vi "IMAQ FPGA Camera Link Pixel Bus to Vision Pixel Bus U32x1.vi"(5 "Reset Overflow":bool, 6 "Ready for Output":bool=TRUE, 7 "Overflow In":bool, 8 "Input Valid":bool=TRUE, 9 "Frame Valid In":bool, 10 "Line Valid In":bool, 11 "Pixel In":u32) -> (0 "Output Valid":bool, 2 "Acquisition Overflow":bool, 3 "Vision Pixel Bus Out":T1)   [LabVIEW 2020]
doc: "The Pixel Bus to Vision Pixel Bus takes the <B>Pixel In</B> and the timing signals (Line Valid, Frame Valid, and Input Valid) and converts them to the data structure used by Vision FPGA functions where the Line Valid and Frame Valid are part of the <B>Vision Pixel Bus Out</B> data structure.\n\nIf Ready For Output is ever False (i.e. downstream VIs are not ready for new pixel data), and this VI is about to output a valid Vision Pixel Bus, the Acquisition Overflow will assert and stay high to indicate pixel data was lost. The CameraLink pixel bus can not be slowed down, so the downstream processing VIs and transfer VIs need to ensure they can handle the CameraLink throughput to avoid missing pixels."
uses:
  <vilib>/visionFPGA/Controls/IMAQ FPGA Pixel Bus RGB32x1.ctl
  <vilib>/visionFPGA/Basics/Camera Link Acquisition/Controls/IMAQ FPGA Camera Link Pixel Bus to Vision Bus State.ctl
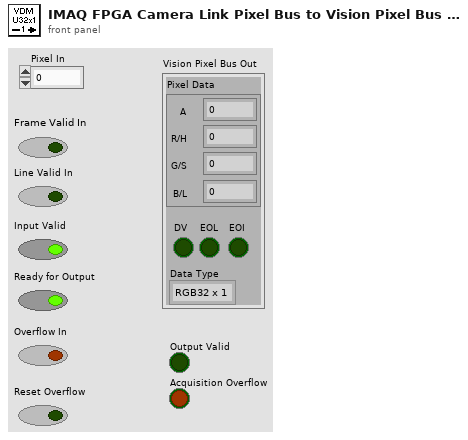
[diagram p1: front panel]
types:
  T1 = typedef "IMAQ FPGA Pixel Bus RGB32x1.ctl" = cluster{"Pixel Data":cluster{"A":u8, "R/H":u8, "G/S":u8, "B/L":u8}, "DV":bool, "EOL":bool, "EOI":bool, "Data Type":enum16{"RGB32 x 1"}}
  T2 = typedef "IMAQ FPGA Camera Link Pixel Bus to Vision Bus State.ctl" = enum16{"WaitForFirstPixel", "WaitForEndOfLine", "WaitForStartofNextLineOrEndOfImage", "HandleEndOfImage"}
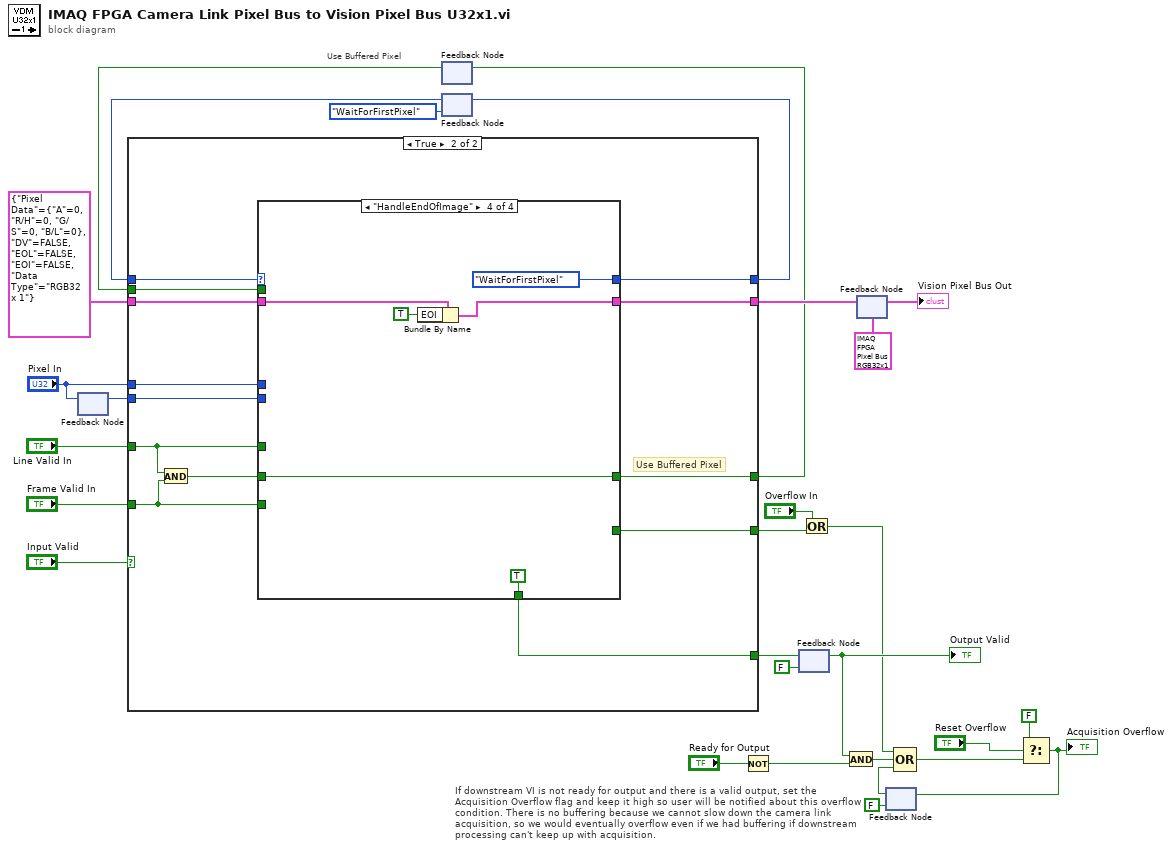
[diagram p0: block diagram]
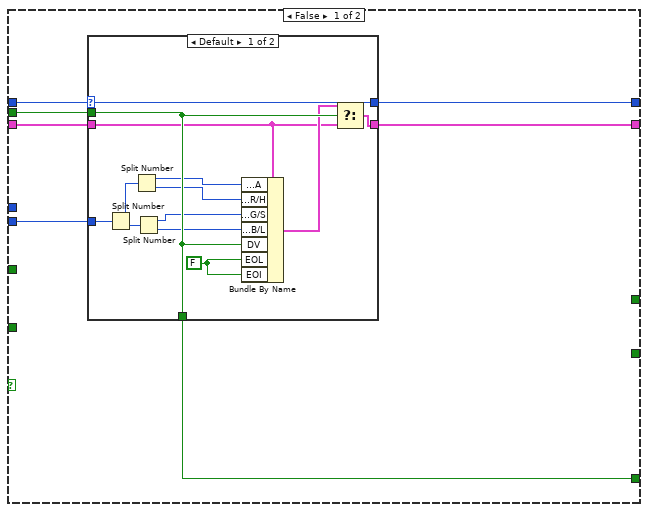
[diagram p2: hidden frame]
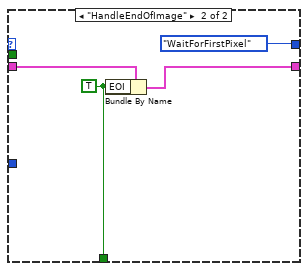
[diagram p3: hidden frame]
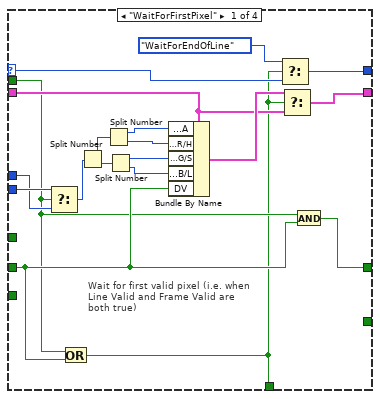
[diagram p4: hidden frame]
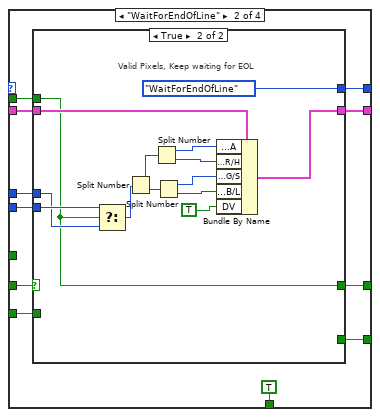
[diagram p5: hidden frame]
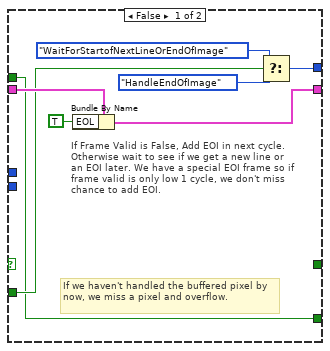
[diagram p6: hidden frame]
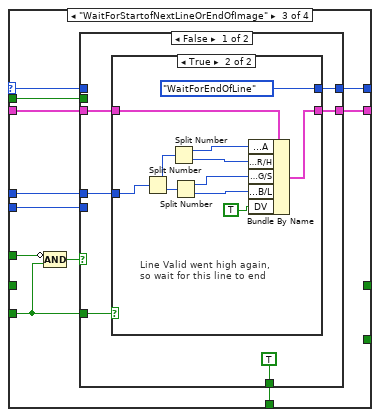
[diagram p7: hidden frame]
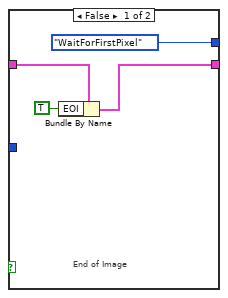
[diagram p8: hidden frame]
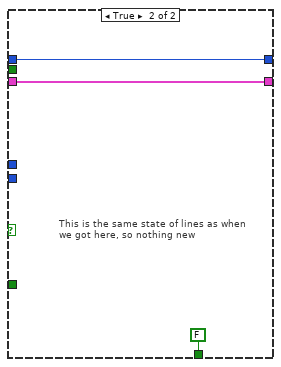
[diagram p9: hidden frame]
diagram:
  # "Use Buffered Pixel"
  # "If downstream VI is not ready for output and there is a valid output, set the Acquisition Overflow flag and keep it high so user will be notified about this overflow condition. There is no buffering because we cannot slow down the camera link acquisition, so we would eventually overflow even if we had buffering if downstream processing can't keep up with acquisition."
  n1 = feedback #1() -> (w7:u32)  [unwired: 1 in]
  n2 = feedback-in #1("Pixel In") -> ()
  n3 = feedback #2() -> (w8:bool)  [unwired: 1 in]
  n4 = feedback #3(IMAQ_FPGA_Camera_Link_Pixel_Bus_to_Vision_Bus_State."WaitForFirstPixel") -> (w11:T2)
  n5 = case shown="True" "Input Valid" {
    tunnel: [w32 w60] -> w25
    tunnel: "Line Valid In" -> [_ w62]
    tunnel: "Frame Valid In" -> [_ w61]
    tunnel: [w34 w65] -> w24
    tunnel: T1 {"Pixel Data"={"A"=0, "R/H"=0, "G/S"=0, "B/L"=0}, "DV"=FALSE, "EOL"=FALSE, "EOI"=FALSE, "Data Type"=enum."RGB32 x 1"} ("Vision Pixel Bus Out") -> [w35 w66]
    tunnel: "Pixel In" -> [_ w64]
    tunnel: [w33 w59] -> w12
    tunnel: w11 -> [w36 w58]
    tunnel: [_ w57] -> w10
    tunnel: w8 -> [w31 w56]
    tunnel: w7 -> [w30 w55]
    tunnel: [_ w54] -> w5
    frame False {
      n6 = case shown="Default" w36 {
        selector: w36 -> [w49 _]
        tunnel: w35 -> [w45 w53]
        tunnel: [w44 w52] -> w34
        tunnel: [w49 IMAQ_FPGA_Camera_Link_Pixel_Bus_to_Vision_Bus_State."WaitForFirstPixel"] -> w33
        tunnel: [w47 w50] -> w32
        tunnel: w31 -> [w47 _]
        tunnel: w30 -> [w43 _]
        frame Default {
          w48 = FALSE ("EOL")
          n7 = Split Number(x=w43) -> (hi(x)=w42:u16, lo(x)=w41:u16)
          n8 = Split Number(x=w42) -> (hi(x)=w39:u8, lo(x)=w40:u8)
          n9 = Split Number(x=w41) -> (hi(x)=w37:u8, lo(x)=w38:u8)
          n10 = Bundle By Name(cluster=w45, "Pixel Data.A"=w39, "Pixel Data.R/H"=w40, "Pixel Data.G/S"=w37, "Pixel Data.B/L"=w38, "DV"=w47, "EOL"=w48, "EOI"=w48) -> (w46:T1)
          n11 = Select(t=w46, s=w47, f=w45) -> (s? t:f=w44:T1)
        }
        frame "HandleEndOfImage" {
          w50 = TRUE ("EOI")
          n12 = Bundle By Name(cluster=w53, "EOI"=w50) -> (w52:T1)
        }
      }
    }
    frame True {
      # "Use Buffered Pixel"
      n13 = And(x=w62, y=w61) -> (x .and. y?=w63:bool)
      n14 = case shown="\"HandleEndOfImage\"" w58 {
        selector: w58 -> [w84 _ w127 _]
        tunnel: [w85 w92 w126 IMAQ_FPGA_Camera_Link_Pixel_Bus_to_Vision_Bus_State."WaitForFirstPixel"] -> w59
        tunnel: w61 -> [_ w91 w122 _]
        tunnel: w62 -> [_ _ w124 _]
        tunnel: w66 -> [w80 w95 w129 w158]
        tunnel: [w83 w93 w128 w156] -> w65
        tunnel: w64 -> [w78 w94 w121 _]
        tunnel: w63 -> [w76 w96 _ w154]
        tunnel: [w74 TRUE w125 TRUE] -> w60
        tunnel: [w77 w87 _ w154] -> w57
        tunnel: w56 -> [w75 w89 w120 _]
        tunnel: w55 -> [w79 w88 w119 _]
        tunnel: [_ w86 _ _] -> w54
        frame "WaitForFirstPixel" {
          # "Wait for first valid pixel (i.e. when Line Valid and Frame Valid are both true)"
          n15 = Select(t=w79, s=w75, f=w78) -> (s? t:f=w71:u32)
          n16 = Or(x=w75, y=w76) -> (x .or. y?=w74:bool)
          n17 = Split Number(x=w71) -> (hi(x)=w73:u16, lo(x)=w72:u16)
          n18 = Split Number(x=w73) -> (hi(x)=w67:u8, lo(x)=w68:u8)
          n19 = Split Number(x=w72) -> (hi(x)=w69:u8, lo(x)=w70:u8)
          n20 = Bundle By Name(cluster=w80, "Pixel Data.A"=w67, "Pixel Data.R/H"=w68, "Pixel Data.G/S"=w69, "Pixel Data.B/L"=w70, "DV"=w76) -> (w81:T1)
          n21 = Select(t=IMAQ_FPGA_Camera_Link_Pixel_Bus_to_Vision_Bus_State."WaitForEndOfLine", s=w74, f=w84) -> (s? t:f=w85:T2)
          n22 = Select(t=w81, s=w74, f=w80) -> (s? t:f=w83:T1)
          n23 = And(x=w75, y=w76) -> (x .and. y?=w77:bool)
        }
        frame "WaitForEndOfLine" {
          n24 = case shown="True" w96 {
            tunnel: w95 -> [w104 w118]
            tunnel: w94 -> [_ w113]
            tunnel: [w103 w117] -> w93
            tunnel: [w98 IMAQ_FPGA_Camera_Link_Pixel_Bus_to_Vision_Bus_State."WaitForEndOfLine"] -> w92
            tunnel: w91 -> [w101 _]
            tunnel: w89 -> [w97 w112]
            tunnel: w88 -> [_ w114]
            tunnel: [_ w112] -> w87
            tunnel: [w97 _] -> w86
            frame False {
              # "If we haven't handled the buffered pixel by now, we miss a pixel and overflow."
              # "If Frame Valid is False, Add EOI in next cycle. Otherwise wait to see if we get a new line or an EOI later. We have a special EOI frame so if frame valid is only low 1 cycle, we don't miss chance to add EOI."
              n25 = Bundle By Name(cluster=w104, "EOL"=TRUE) -> (w103:T1)
              n26 = Select(t=IMAQ_FPGA_Camera_Link_Pixel_Bus_to_Vision_Bus_State."WaitForStartofNextLineOrEndOfImage", s=w101, f=IMAQ_FPGA_Camera_Link_Pixel_Bus_to_Vision_Bus_State."HandleEndOfImage") -> (s? t:f=w98:T2)
            }
            frame True {
              # "Valid Pixels, Keep waiting for EOL"
              n27 = Select(t=w114, s=w112, f=w113) -> (s? t:f=w109:u32)
              n28 = Split Number(x=w109) -> (hi(x)=w111:u16, lo(x)=w110:u16)
              n29 = Split Number(x=w111) -> (hi(x)=w108:u8, lo(x)=w107:u8)
              n30 = Split Number(x=w110) -> (hi(x)=w105:u8, lo(x)=w106:u8)
              n31 = Bundle By Name(cluster=w118, "Pixel Data.A"=w108, "Pixel Data.R/H"=w107, "Pixel Data.G/S"=w105, "Pixel Data.B/L"=w106, "DV"=TRUE) -> (w117:T1)
            }
          }
        }
        frame "WaitForStartofNextLineOrEndOfImage" {
          n32 = Compound Arithmetic op=AND(invert w124, w122) -> (w123:bool)
          n33 = case shown="False" w123 {
            tunnel: w129 -> [w134 w152]
            tunnel: [w133 w152] -> w128
            tunnel: w127 -> [_ w153]
            tunnel: [w132 w153] -> w126
            tunnel: [TRUE FALSE] -> w125
            tunnel: w122 -> [w131 _]
            tunnel: w121 -> [w130 _]
            tunnel: w120 -> [_ _]
            tunnel: w119 -> [_ _]
            frame False {
              n34 = case shown="True" w131 {
                tunnel: w134 -> [w139 w149]
                tunnel: [w137 w148] -> w133
                tunnel: [IMAQ_FPGA_Camera_Link_Pixel_Bus_to_Vision_Bus_State."WaitForFirstPixel" IMAQ_FPGA_Camera_Link_Pixel_Bus_to_Vision_Bus_State."WaitForEndOfLine"] -> w132
                tunnel: w130 -> [_ w144]
                frame False {
                  # "End of Image"
                  n35 = Bundle By Name(cluster=w139, "EOI"=TRUE) -> (w137:T1)
                }
                frame True {
                  # "Line Valid went high again, so wait for this line to end"
                  n36 = Split Number(x=w144) -> (hi(x)=w146:u16, lo(x)=w145:u16)
                  n37 = Split Number(x=w146) -> (hi(x)=w140:u8, lo(x)=w141:u8)
                  n38 = Split Number(x=w145) -> (hi(x)=w142:u8, lo(x)=w143:u8)
                  n39 = Bundle By Name(cluster=w149, "Pixel Data.A"=w140, "Pixel Data.R/H"=w141, "Pixel Data.G/S"=w142, "Pixel Data.B/L"=w143, "DV"=TRUE) -> (w148:T1)
                }
              }
            }
            frame True {
              # "This is the same state of lines as when we got here, so nothing new"
            }
          }
        }
        frame "HandleEndOfImage" {
          n40 = Bundle By Name(cluster=w158, "EOI"=TRUE) -> (w156:T1)
        }
      }
    }
  }
  n41 = feedback-in #2(w10) -> ()
  n42 = feedback-in #3(w12) -> ()
  n43 = Not(x="Ready for Output") -> (.not. x?=w22:bool)
  n44 = feedback #4(FALSE) -> (w21:bool)
  "Output Valid" <- w21
  n45 = feedback-in #4(w25) -> ()
  n46 = Or(x="Overflow In", y=w5) -> (x .or. y?=w4:bool)
  n47 = And(x=w21, y=w22) -> (x .and. y?=w20:bool)
  n48 = feedback #5(T1 {"Pixel Data"={"A"=0, "R/H"=0, "G/S"=0, "B/L"=0}, "DV"=FALSE, "EOL"=FALSE, "EOI"=FALSE, "Data Type"=enum."RGB32 x 1"} ("Vision Pixel Bus Out")) -> (→"Vision Pixel Bus Out":T1)
  n49 = feedback-in #5(w24) -> ()
  n50 = feedback #6(FALSE) -> (w19:bool)
  n51 = Compound Arithmetic op=OR(w4, w20, w19) -> (w16:bool)
  n52 = Select(t=FALSE, s="Reset Overflow", f=w16) -> (s? t:f=w15:bool)
  "Acquisition Overflow" <- w15
  n53 = feedback-in #6(w15) -> ()
